vi "Create from Node-ID.vi"(7 "Function Code":T1 items=["NMT"=0, "EMCY/SYNC"=1, "TIME"=2, "PDO1 (tx)"=3, "PDO1 (rx)"=4, "PDO2 (tx)"=5, "PDO2 (rx)"=6, "PDO3 (tx)"=7, "PDO3 (rx)"=8, "PDO4 (tx)"=9, "PDO4 (rx)"=10, "SDO (tx)"=11, "SDO (rx)"=12, "NMT error control"=14], 9 "Data":u8[](array[numeric]) format="%.0x", 10 "Node-ID":u8) -> (3 "CANopen Message":refnum<class "CANopen Message.lvclass">)   [LabVIEW 2020, in "CANopen.lvlib" / "CANopen Message.lvclass"]
uses:
  CANopen Message.lvclass
  CANopen Message.lvclass/CANopen Message.ctl
  Typedefs/Function Code.ctl
  CANopen.lvlib
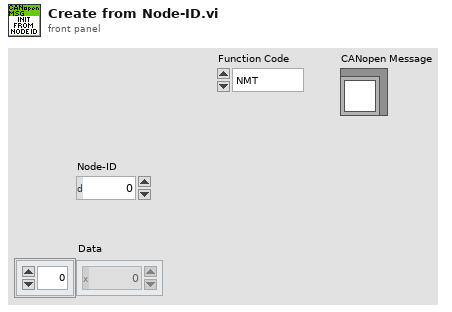
[diagram p1: front panel]
types:
  T1 = typedef "CANopen.lvlib/Function Code.ctl" = u8
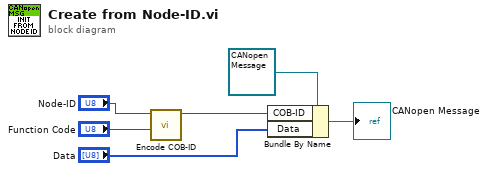
[diagram p0: block diagram]
diagram:
  n1 = call "Encode COB-ID.vi"("Function code"="Function Code", "Node-ID"="Node-ID") -> ("COD-ID"=w3:u32)  [unwired: 9 in]
  n2 = Bundle By Name(cluster=refnum<class "CANopen Message.lvclass"> refnum ("CANopen Message out"), "COB-ID"=w3, "Data"="Data") -> (→"CANopen Message":refnum<class "CANopen Message.lvclass">)
